vi "MASTER DEMO.vi"() -> ()   [LabVIEW 2019]
uses:
  <userlib>/Onshape/_SubVI/EdgeDetect_Camera.vi
  <userlib>/Onshape/_SubVI/z did wid and eid.vi
panel:
  out "SVG":picture
  in  "stop":bool
  out "Image":picture
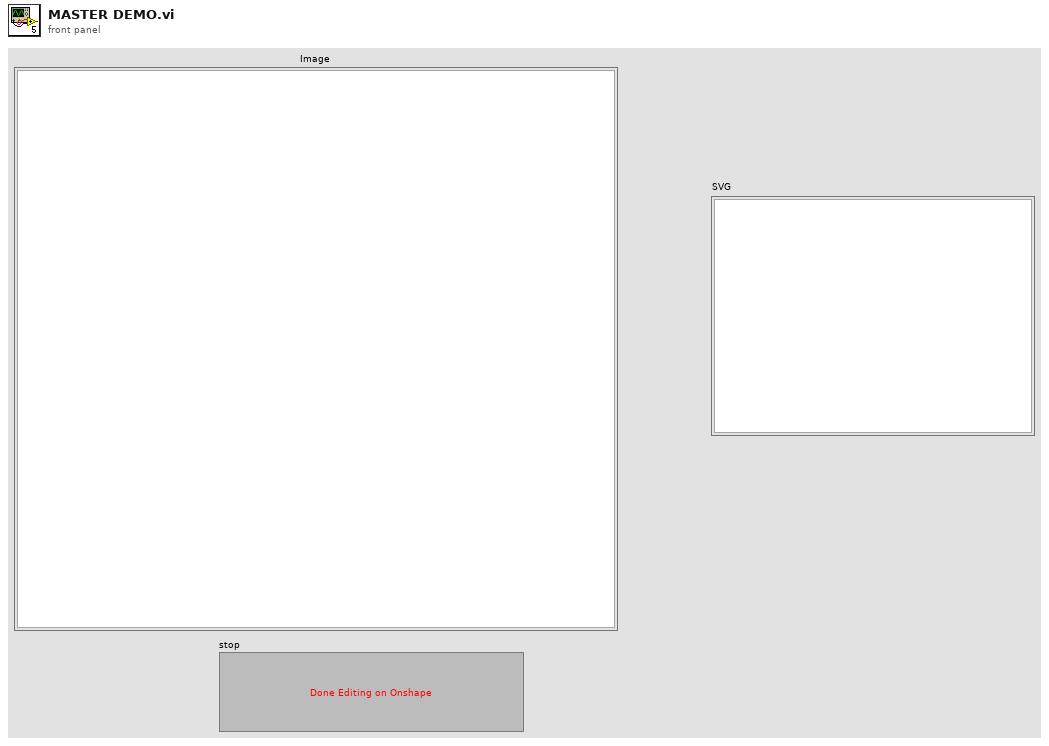
[diagram p1: front panel]
types:
  T1 = typedef "Cluster.ctl" = cluster{"Date":string, "On-Nonce":string, "eid":string, "wid":string, "did":string, "name":string, "method":string, "Accept":string, "User-Agent":string, "Content-Type":string, "stack":string, "headers":string[], "payload":string, "addition":string, "path":string, "Authorization":string, "secret_key":string, "access_key":string}
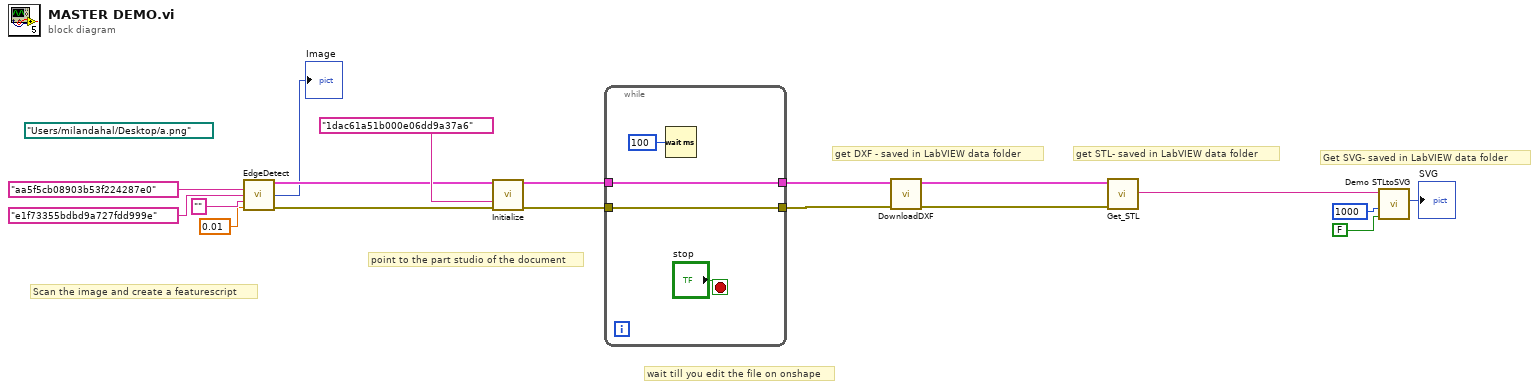
[diagram p0: block diagram]
diagram:
  (unwired) path "/Users/milandahal/Desktop/a.png" ("Image Path")
  # "wait till you edit the file on onshape"
  # "Get SVG- saved in LabVIEW data folder"
  # "get DXF - saved in LabVIEW data folder"
  # "get STL- saved in LabVIEW data folder"
  # "point to the part studio of the document"
  # "Scan the image and create a featurescript"
  n1 = call-poly <userlib>:"EdgeDetect.vi"("did"="aa5f5cb08903b53f224287e0", "wid"="e1f73355bdbd9a727fdd999e", "eid"="", "Scaling Factor"=0.01) -> ("Device Out"=w11:T1, "image 2"=→"Image":picture, "error out"=w9:errorcluster)  [unwired: 8 in, 1 out]
  n2 = call-poly <userlib>:"Initialize.vi"("Device In"=w11, "eid"="1dac61a51b000e06dd9a37a6", "error in"=w9) -> ("Device Out"=w8:T1, "error out"=w6:errorcluster)  [unwired: 11 in]
  n3 = while {
    tunnel: w8 -> [w20]
    tunnel: [w20] -> w7
    tunnel: w6 -> [w19]
    tunnel: [w19] -> w5
    stop <- "stop" stop-if-true
    n4 = Wait (ms)(milliseconds to wait=u32 100) -> ()  [unwired: 1 out]
  }
  n5 = call <userlib>:"DownloadDXF.vi"("error in"=w5, "Device In"=w7) -> ("error out"=w1:errorcluster, "Device Out"=w2:T1)  [unwired: 6 in, 2 out]
  n6 = call <userlib>:"Get_STL.vi"("error in"=w1, "Device In"=w2) -> ("stl text"=w10:string)  [unwired: 6 in, 3 out]
  n7 = call <userlib>:"Demo STLtoSVG.vi"("File True/ String False"=FALSE, "Scale"=1000, "STL String"=w10) -> ("new picture"=→"SVG":picture)  [unwired: 8 in]
